vi "2.2 Waypoint Monitor.vi"(8 "Error In":errorcluster, 11 "Waypoint Queue In":T4) -> (0 "Error Out":errorcluster, 1 "Waypoint Valid?":bool, 2 "Current Waypoint":T1, 3 "Waypoint Queue Out":T4)   [LabVIEW 2011]
doc: "TODO: important As of 10/27 this VI only works for the Drive option\n\nWaypoint Monitor takes two things from the global variable - the list of waypoints and\nthe position of the robot at the time.\n\nIt compares the current position to the position of the current waypoint, and if that distance\nis less than the required accuracy the current waypoint value is incremented"
uses:
  2x3-RIO-OCU Comm/2x3 Typedefs/waypointQueue.ctl
  2x3-RIO-OCU Comm/2x3 Typedefs/ocuWaypoint.ctl
  2x3-RIO-OCU Comm/2x3 Typedefs/waypointTypes.ctl
  2 Typedefs/UTM Location.ctl
  2 Globals/2 Global.vi
panel:
  # "Waypoint Monitor takes one thing from the global variable -\nthe position of the robot at the time.\n\nIt compares the current position to the position of the current waypoint, and if that distance\nis less than the required accuracy the current waypoint is removed from the queue of\nwaypoints.\n\nTODO - Round cases"
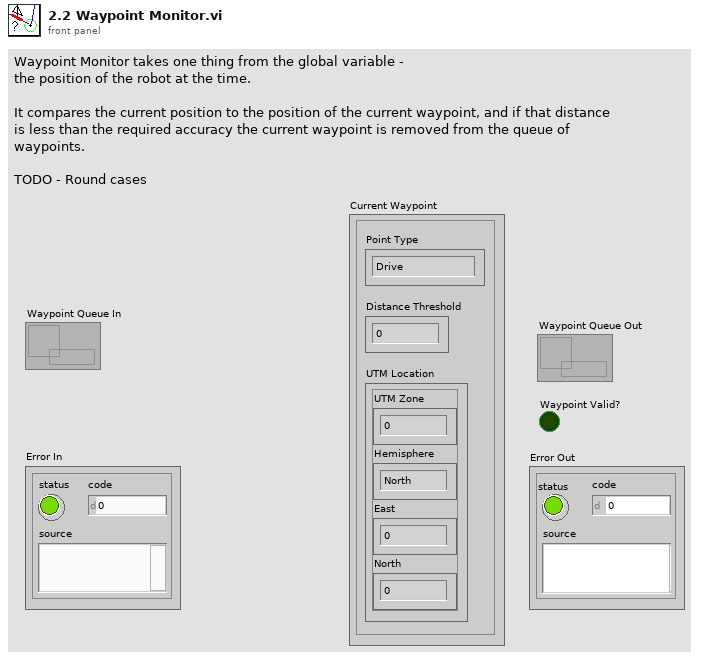
[diagram p1: front panel]
types:
  T1 = typedef "ocuWaypoint.ctl" = cluster{"Point Type":T2, "Distance Threshold":dbl, "UTM Location":T3}
  T2 = typedef "waypointTypes.ctl" = enum16{"Drive", "Round Port", "Round Starboard", "Stay"}
  T3 = typedef "UTM Location.ctl" = cluster{"UTM Zone":dbl, "Hemisphere":enum16{"North", "South"}, "East":dbl, "North":dbl}
  T4 = typedef "waypointQueue.ctl" = refnum<queue>
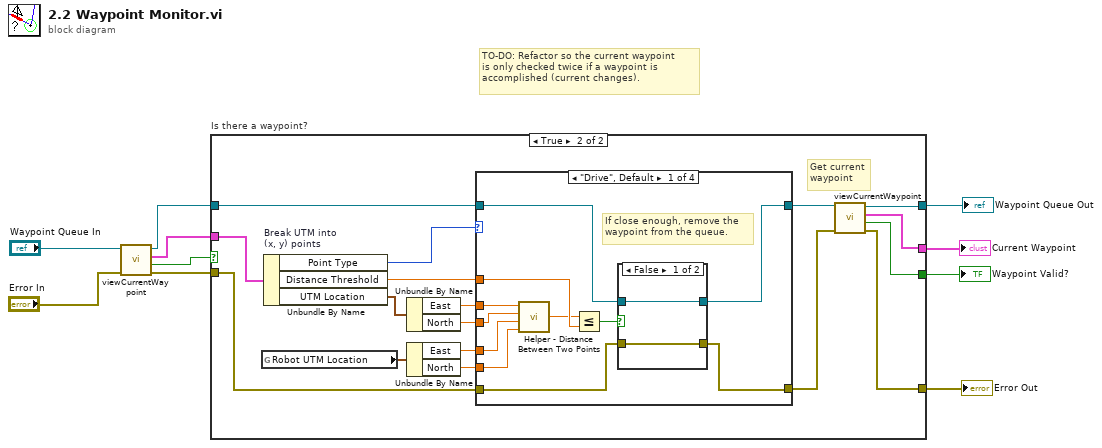
[diagram p0: block diagram]
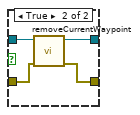
[diagram p3: hidden frame]
diagram:
  # "TO-DO: Refactor so the current waypoint\nis only checked twice if a waypoint is\naccomplished (current changes)."
  n1 = call "viewCurrentWaypoint.vi"("Error In"="Error In", "Waypoint Queue In"="Waypoint Queue In") -> ("Error Out"=w6:errorcluster, "Waypoint Valid?"=w9:bool, "Current Waypoint"=w7:T1, "Waypoint Queue Out"=w8:T4)  [unwired: 6 in]
  n2 = case "Is there a waypoint?" shown="True" w9 {
    selector: w9 -> [w11 _]
    tunnel: w8 -> [w14 w22]
    tunnel: w7 -> [w12 w31]
    tunnel: w6 -> [w13 w21]
    tunnel: [w14 w17] -> w4
    tunnel: [w13 w18] -> w3
    tunnel: [w12 w16] -> w1
    tunnel: [w11 w15] -> w2
    frame False {
    }
    frame True {
      # "Get current\nwaypoint"
      n3 = global read "2 Global.vi" "Robot UTM Location"() -> (w28:T3)
      n4 = Unbundle By Name "Break UTM into\n(x, y) points"(w31) -> ("Point Type"=w30:T2, "Distance Threshold"=w23:dbl, "UTM Location"=w29:T3)
      n5 = Unbundle By Name(w29) -> ("East"=w27:dbl, "North"=w26:dbl)
      n6 = Unbundle By Name(w28) -> ("East"=w25:dbl, "North"=w24:dbl)
      n7 = case shown="\"Drive\", Default" w30 {
        tunnel: w27 -> [w42 _ _ _]
        tunnel: w26 -> [w41 _ _ _]
        tunnel: w25 -> [w40 _ _ _]
        tunnel: w24 -> [w39 _ _ _]
        tunnel: w23 -> [w38 _ _ _]
        tunnel: w22 -> [w35 w50 w52 w54]
        tunnel: w21 -> [w34 w49 w51 w53]
        tunnel: [w33 w49 w51 w53] -> w19
        tunnel: [w32 w50 w52 w54] -> w20
        frame "Drive", Default {
          # "If close enough, remove the\nwaypoint from the queue."
          n8 = call "Helper - Distance Between Two Points.vi"("y 2"=w39, "x 2"=w40, "y"=w41, "x"=w42) -> ("Numeric"=w37:dbl)
          n9 = Less Or Equal?(x=w37, y=w38) -> (x <= y?=w36:bool)
          n10 = case shown="False" w36 {
            tunnel: w35 -> [w43 w48]
            tunnel: w34 -> [w44 w47]
            tunnel: [w44 w46] -> w33
            tunnel: [w43 w45] -> w32
            frame False {
            }
            frame True {
              n11 = call "removeCurrentWaypoint.vi"("Error In"=w47, "Waypoint Queue In"=w48) -> ("Error Out"=w46:errorcluster, "Waypoint Queue Out"=w45:T4)  [unwired: 7 in, 1 out]
            }
          }
        }
        frame "Round Port" {
          # "Not yet implemented"
        }
        frame "Round Starboard" {
          # "Not yet implemented"
        }
        frame "Stay" {
        }
      }
      n12 = call "viewCurrentWaypoint.vi"("Error In"=w19, "Waypoint Queue In"=w20) -> ("Error Out"=w18:errorcluster, "Waypoint Valid?"=w15:bool, "Current Waypoint"=w16:T1, "Waypoint Queue Out"=w17:T4)  [unwired: 6 in]
    }
  }
  "Waypoint Queue Out" <- w4
  "Error Out" <- w3
  "Waypoint Valid?" <- w2
  "Current Waypoint" <- w1
